vi "test Import To Empty Module Same Slot.vi"(8 "error in (no error)":errorcluster, 11 "TestCase in":refnum<class "SLSC Switch Import Export Unit Tests.lvclass">) -> (0 "error out":errorcluster, 3 "TestCase out":refnum<class "SLSC Switch Import Export Unit Tests.lvclass">)   [LabVIEW 2017, in "SLSC Switch Import Export Unit Tests.lvclass"]
uses:
  SLSC Switch Import Export Unit Tests.lvclass
  <vilib>/addons/_JKI Toolkits/VI Tester/TestCase.llb/TestCase.lvclass
  <vilib>/NI/NI VeriStand Custom Device Import and Export Tool/ImportExport.lvlib
  Scripting/NI-SWITCH Scripting.lvlib
  Shared/VeriStand System Definition Test Utilities/VeriStand System Definition Test Utilities.lvlib
  Shared/Endpoint Configuration Enum.ctl
  Shared/NI-SWITCH Shared.lvlib
  Shared/Endpoint Configuration Cluster.ctl
  C:/Program Files (x86)/National Instruments/LabVIEW 2017/vi.lib/addons/_JKI Toolkits/VI Tester/TestCase.llb/TestCase.lvclass
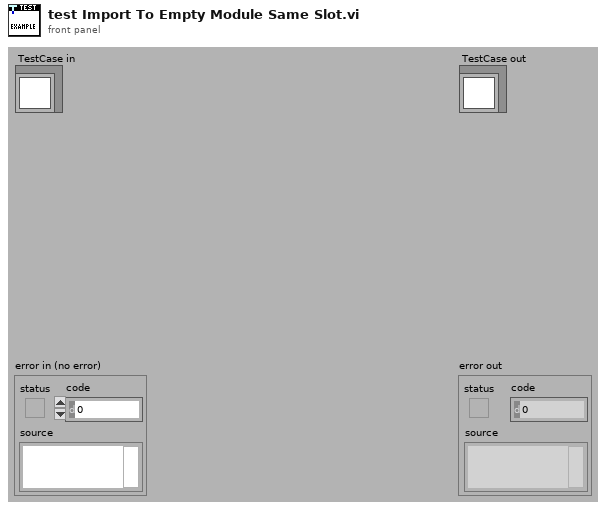
[diagram p1: front panel]
types:
  T1 = cluster{"Ignore Properties":string[], "Ignore Top Level Name":bool}
  T2 = typedef "NI-SWITCH Shared.lvlib/Endpoint Configuration Cluster.ctl" = cluster{"Endpoint":string, "Configuration":T3}
  T3 = typedef "NI-SWITCH Shared.lvlib/Endpoint Configuration Enum.ctl" = enum16{"Load", "Source", "Configuration"}
  T4 = typedef "Custom Device API.lvlib/Custom Device Item Ref.ctl" = u64
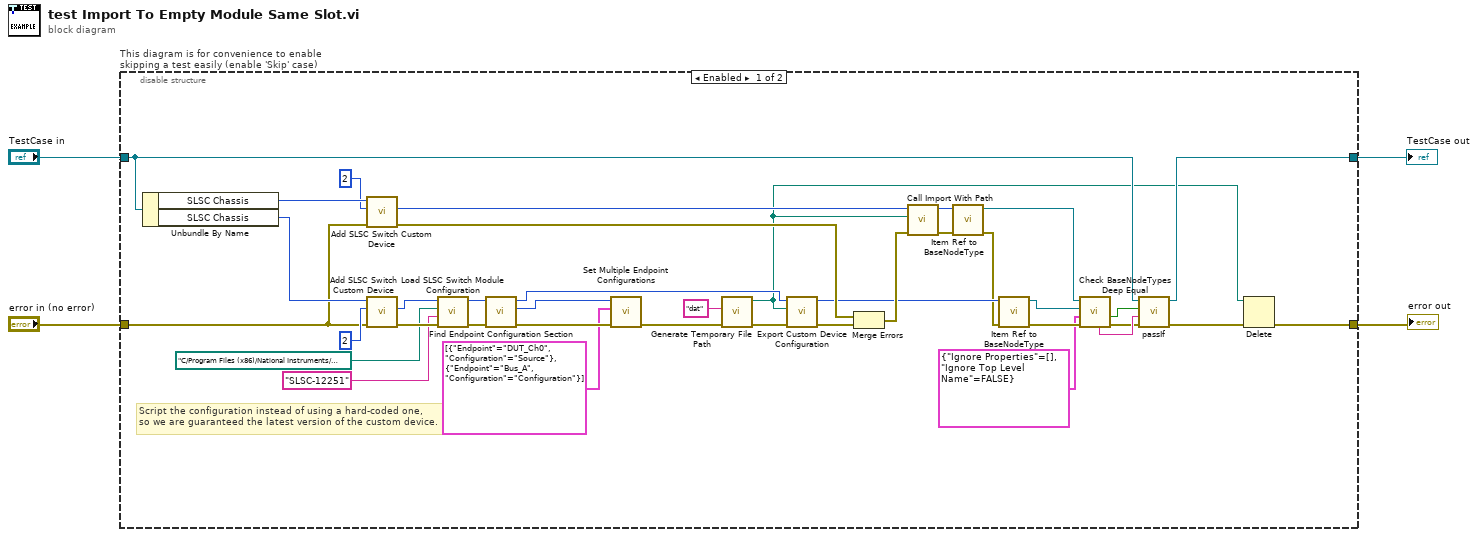
[diagram p0: block diagram]
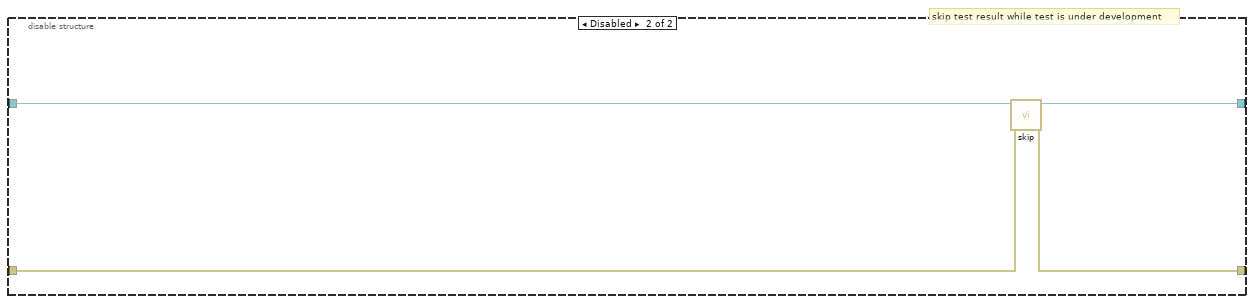
[diagram p2: hidden frame]
diagram:
  n1 = disable-structure "This diagram is for convenience to enable skipping a test easily (enable 'Skip' case)" shown="Enabled" {
    disable-tunnel: "TestCase in" -> [w29 w46]
    disable-tunnel: [w8 w44] -> w1
    disable-tunnel: [w6 w45] -> w3
    disable-tunnel: "error in (no error)" -> [w23 w43]
    frame Enabled {
      # "Script the configuration instead of using a hard-coded one,\nso we are guaranteed the latest version of the custom device."
      n2 = Unbundle By Name(w29) -> ("SLSC Chassis"=w24:u64, "SLSC Chassis"=w42:u64)
      n3 = call "Add SLSC Switch Custom Device.vi"("error in"=w23, "slot number"=u32 2, "slsc chassis in"=w24) -> ("error out"=w37:errorcluster, "slsc switch custom device"=w9:T4)  [unwired: 6 in, 1 out]
      n4 = call "Add SLSC Switch Custom Device.vi"("error in"=w23, "slot number"=u32 2, "slsc chassis in"=w42) -> ("error out"=w22:errorcluster, "slsc switch custom device"=w20:T4)  [unwired: 6 in, 1 out]
      n5 = call "Load SLSC Switch Module Configuration.vi"("error in"=w22, "product name"="SLSC-12251", "switches json file"=path "C:/Program Files (x86)/National Instruments/Shared/NI-SLSC Switch/Modules/SLSC-12251-switches.json", "slsc switch custom device in"=w20) -> ("error out"=w21:errorcluster, "slsc switch custom device out"=w16:T4)  [unwired: 6 in]
      n6 = call "Find Endpoint Configuration Section.vi"("error in"=w21, "slsc switch custom device in"=w16) -> ("error out"=w17:errorcluster, "endpoint configuration"=w14:T4, "slsc switch custom device out"=w13:T4)  [unwired: 7 in]
      n7 = call "Set Multiple Endpoint Configurations.vi"("error in"=w17, "endpoint configurations"=T2[] [{"Endpoint"="DUT_Ch0", "Configuration"=enum."Source"}, {"Endpoint"="Bus_A", "Configuration"=enum."Configuration"}], "endpoint configuration in"=w14) -> ("error out"=w15:errorcluster)  [unwired: 7 in, 1 out]
      n8 = call <vilib>:"Generate Temporary File Path.vi"("error in (no error)"=w15, "Temporary File Extension (tmp)"="dat") -> ("error out"=w39:errorcluster, "Unique Temporary File Path"=w5:path)  [unwired: 8 in]
      n9 = call <vilib>:"Export Custom Device Configuration.vi"("error in (no error)"=w39, "Path"=w5, "ID"=w13) -> ("error out"=w38:errorcluster, "ID out"=w34:u64)  [unwired: 7 in]
      n10 = Merge Errors(w37, w38) -> (w36:errorcluster)
      n11 = call "Call Import With Path.vi"("error in (no error)"=w36, "Path"=w5, "Node Ptr"=w9) -> ("error out"=w33:errorcluster, "Node Ptr out"=w35:u64)  [unwired: 7 in]
      n12 = call "Item Ref to BaseNodeType.vi"("error in (no error)"=w33, "Item Ref"=w35) -> ("error out"=w32:errorcluster, "BaseNodeType"=w26:refnum<k24>)  [unwired: 8 in]
      n13 = call "Item Ref to BaseNodeType.vi"("error in (no error)"=w32, "Item Ref"=w34) -> ("error out"=w31:errorcluster, "BaseNodeType"=w30:refnum<k24>)  [unwired: 8 in]
      n14 = call "Check BaseNodeTypes Deep Equal.vi"("error in (no error)"=w31, "Settings"=T1 {"Ignore Properties"=[], "Ignore Top Level Name"=FALSE}, "BaseNodeType 2"=w30, "BaseNodeType 1"=w26) -> ("error out"=w25:errorcluster, "Equal?"=w28:bool, "Inequality context"=w27:string)  [unwired: 3 in, 2 out]
      n15 = call-dynamic "passIf.vi"("error in (no error)"=w25, "message (\"\")"=w27, "pass"=w28, "TestCase in"=w29) -> ("error out"=w7:errorcluster, "TestCase out"=w8:refnum<class "SLSC Switch Import Export Unit Tests.lvclass">)  [unwired: 6 in]
      n16 = Delete(path (use dialog)=w5, error in=w7) -> (error out=w6:errorcluster)  [unwired: 3 in, 2 out]
    }
    frame Disabled {
      # "skip test result while test is under development"
      n17 = call <vilib>:"skip.vi"("error in (no error)"=w43, "TestCase in"=w46) -> ("error out"=w45:errorcluster, "TestCase out"=w44:refnum<class "SLSC Switch Import Export Unit Tests.lvclass">)  [unwired: 8 in]
    }
  }
  "error out" <- w3
  "TestCase out" <- w1
